vi "Page_Advanced_Initialize.vi"(6 "ctl references":T1, 8 "error in (no error)":errorcluster, 11 "AB_SourceDistribution in":refnum<class "AB_WebService.lvclass">) -> (0 "error out":errorcluster, 3 "AB_SourceDistribution out":refnum<class "AB_WebService.lvclass">)   [LabVIEW 2020, in "AB_WebService.lvclass"]
uses:
  <vilib>/AppBuilder/AB_Classes/WebService/AB_WebService.lvclass
  <resource>/Framework/Providers/Builds/AppBuilder/AB_UI_Page_Advanced_References.ctl
  <vilib>/AppBuilder/AB_Classes/TargetFile/AB_Targetfile.lvclass
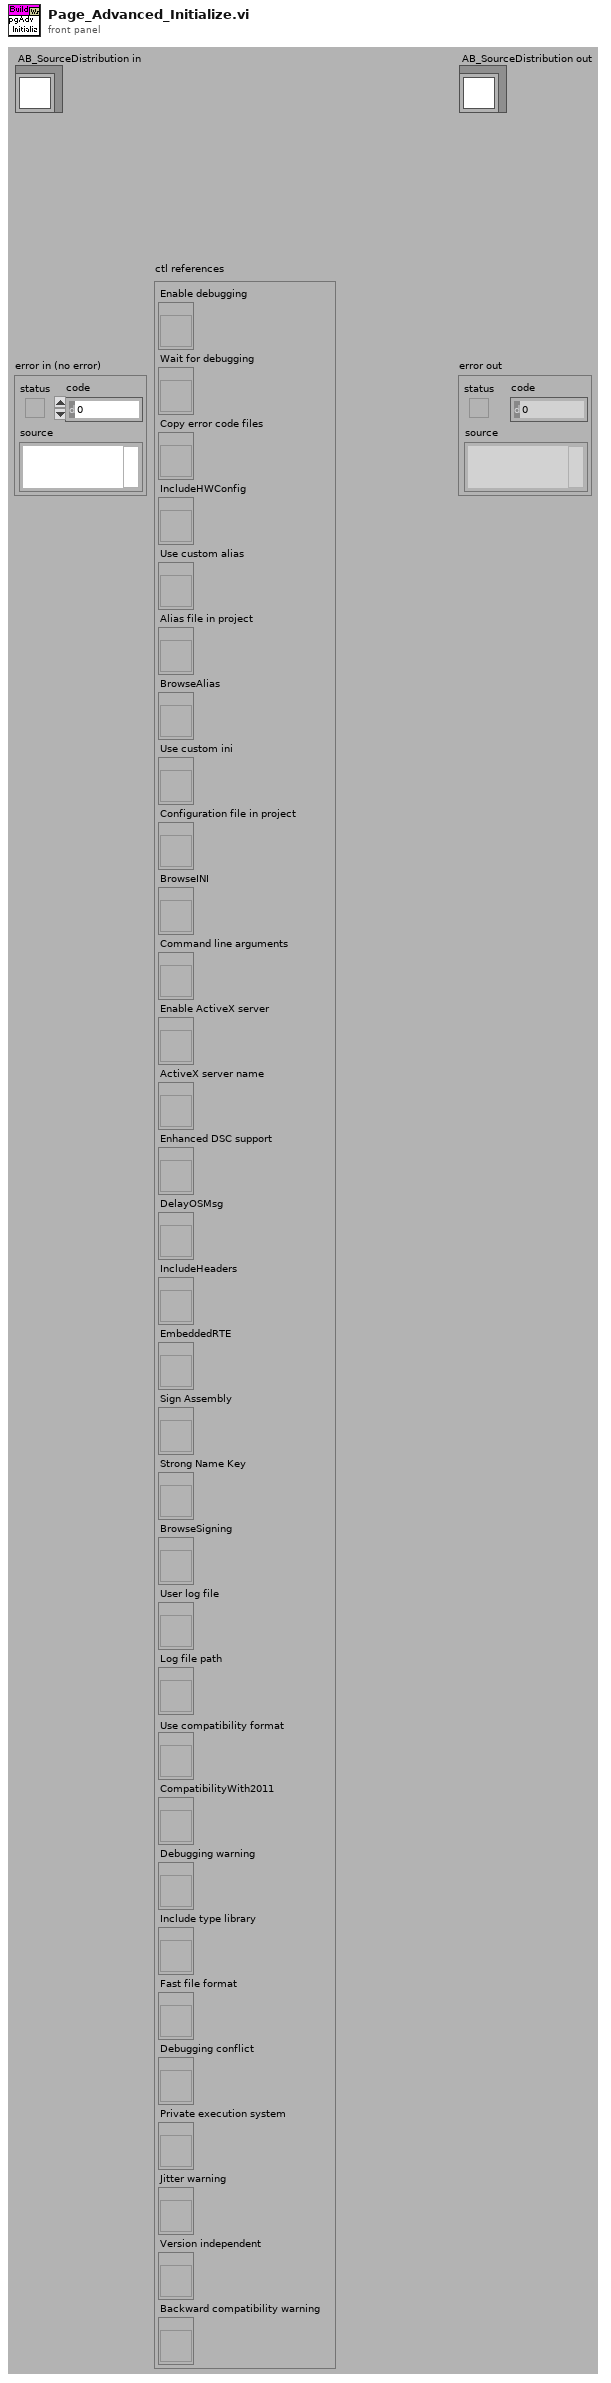
[diagram p1: front panel]
types:
  T1 = typedef "AB_UI_Page_Advanced_References.ctl" = cluster{"Enable debugging":refnum<vi>, "Wait for debugging":refnum<vi>, "Copy error code files":refnum<vi>, "IncludeHWConfig":refnum<vi>, "Use custom alias":refnum<vi>, "Alias file in project":refnum<vi>, "BrowseAlias":refnum<vi>, "Use custom ini":refnum<vi>, "Configuration file in project":refnum<vi>, "BrowseINI":refnum<vi>, "Command line arguments":refnum<vi>, "Enable ActiveX server":refnum<vi>, "ActiveX server name":refnum<vi>, "Enhanced DSC support":refnum<vi>, "DelayOSMsg":refnum<vi>, "IncludeHeaders":refnum<vi>, "EmbeddedRTE":refnum<vi>, "Sign Assembly":refnum<vi>, "Strong Name Key":refnum<vi>, "BrowseSigning":refnum<vi>, "User log file":refnum<vi>, "Log file path":refnum<vi>, "Use compatibility format":refnum<vi>, "CompatibilityWith2011":refnum<vi>, "Debugging warning":refnum<vi>, "Include type library":refnum<vi>, "Fast file format":refnum<vi>, "Debugging conflict":refnum<vi>, "Private execution system":refnum<vi>, "Jitter warning":refnum<vi>, "Version independent":refnum<vi>, "Backward compatibility warning":refnum<vi>}
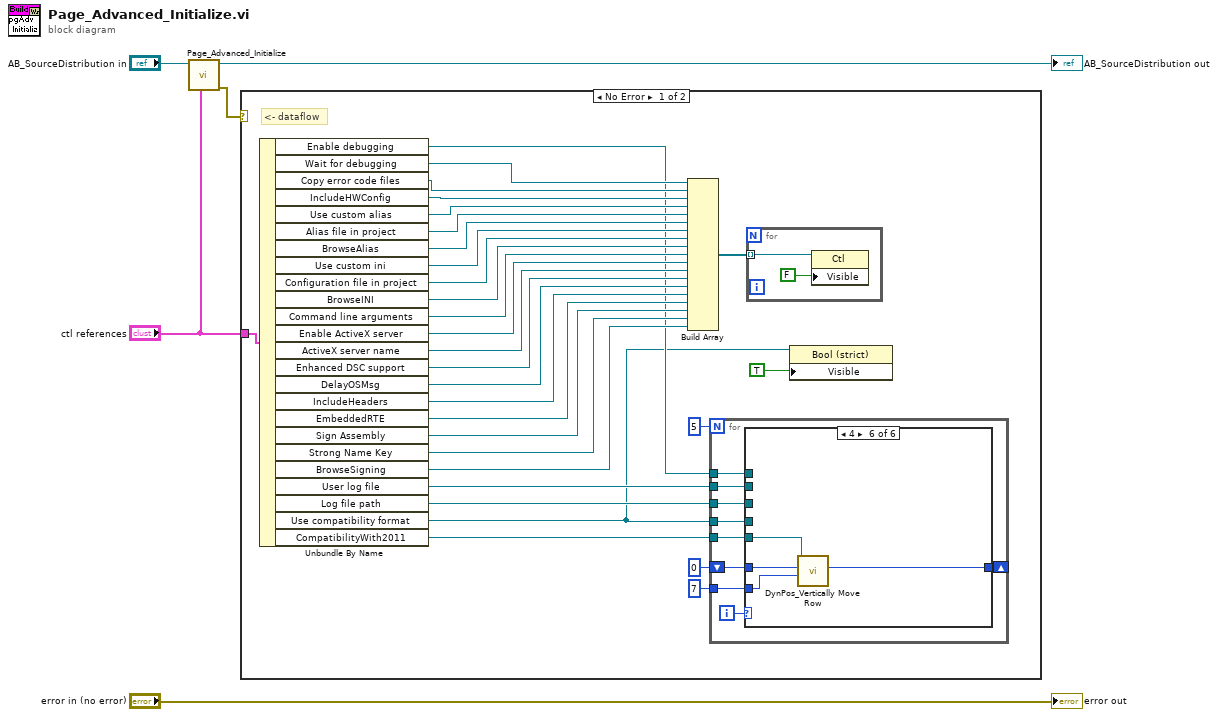
[diagram p0: block diagram]
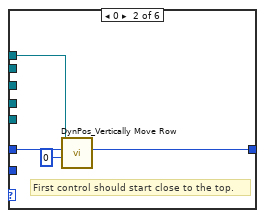
[diagram p3: hidden frame]
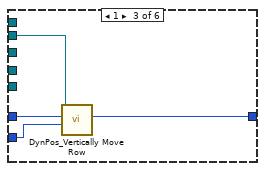
[diagram p4: hidden frame]
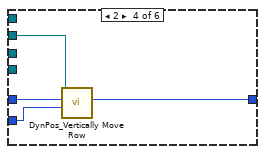
[diagram p5: hidden frame]
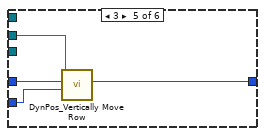
[diagram p6: hidden frame]
diagram:
  n1 = call-parent "Page_Advanced_Initialize.vi"("ctl references"="ctl references", "AB_Build in"="AB_SourceDistribution in") -> ("error out"=w1:errorcluster, "AB_Build out"=→"AB_SourceDistribution out":refnum<class "AB_WebService.lvclass">)  [unwired: 1 in, 7 out]
  n2 = case shown="No Error" w1 {
    tunnel: "ctl references" -> [w35 _]
    frame No Error {
      # "<- dataflow"
      n3 = Unbundle By Name(w35) -> ("Enable debugging"=w9:refnum<vi>, "Wait for debugging"=w34:refnum<vi>, "Copy error code files"=w33:refnum<vi>, "IncludeHWConfig"=w32:refnum<vi>, "Use custom alias"=w31:refnum<vi>, "Alias file in project"=w30:refnum<vi>, "BrowseAlias"=w29:refnum<vi>, "Use custom ini"=w28:refnum<vi>, "Configuration file in project"=w27:refnum<vi>, "BrowseINI"=w26:refnum<vi>, "Command line arguments"=w25:refnum<vi>, "Enable ActiveX server"=w24:refnum<vi>, "ActiveX server name"=w23:refnum<vi>, "Enhanced DSC support"=w22:refnum<vi>, "DelayOSMsg"=w20:refnum<vi>, "IncludeHeaders"=w19:refnum<vi>, "EmbeddedRTE"=w18:refnum<vi>, "Sign Assembly"=w17:refnum<vi>, "Strong Name Key"=w16:refnum<vi>, "BrowseSigning"=w15:refnum<vi>, "User log file"=w13:refnum<vi>, "Log file path"=w12:refnum<vi>, "Use compatibility format"=w7:refnum<vi>, "CompatibilityWith2011"=w6:refnum<vi>)
      n4 = Build Array(w34, w33, w32, w31, w30, w29, w28, w27, w26, w25, w24, w23, w22, w20, w19, w18, w17, w16, w15) -> (w21:refnum<vi>[])
      n5 = for {
        N: 5 -> [_]
        tunnel: w13 -> [w43]
        tunnel: w12 -> [w42]
        shift-right: [w41] -> _
        shift-left: 0 ("Bottom pixel") -> [w40]
        tunnel: 7 ("Bottom pixel") -> [w39]
        tunnel: w9 -> [w38]
        tunnel: w7 -> [w37]
        tunnel: w6 -> [w36]
        i -> [w44]
        n6 = case shown="4" w44 {
          tunnel: w43 -> [_ _ w50 _ _ _]
          tunnel: w42 -> [_ _ _ w54 _ _]
          tunnel: [w45 w48 w53 w57 w61 w65] -> w41
          tunnel: w40 -> [w45 w47 w52 w56 w60 w64]
          tunnel: w39 -> [_ _ w51 w55 w59 w63]
          tunnel: w38 -> [_ w46 _ _ _ _]
          tunnel: w37 -> [_ _ _ _ w58 _]
          tunnel: w36 -> [_ _ _ _ _ w62]
          frame Default {
          }
          frame 0 {
            # "First control should start close to the top."
            n7 = call <vilib>:"DynPos_Vertically Move Row.vi"("Pixel separation (6)"=0, "Bottom of last control"=w47, "Control"=w46) -> ("Bottom pixel"=w48:i32)  [unwired: 1 in, 7 out]
          }
          frame 1 {
            n8 = call <vilib>:"DynPos_Vertically Move Row.vi"("Pixel separation (6)"=w51, "Bottom of last control"=w52, "Control"=w50) -> ("Bottom pixel"=w53:i32)  [unwired: 1 in, 7 out]
          }
          frame 2 {
            n9 = call <vilib>:"DynPos_Vertically Move Row.vi"("Pixel separation (6)"=w55, "Bottom of last control"=w56, "Control"=w54) -> ("Bottom pixel"=w57:i32)  [unwired: 1 in, 7 out]
          }
          frame 3 {
            n10 = call <vilib>:"DynPos_Vertically Move Row.vi"("Pixel separation (6)"=w59, "Bottom of last control"=w60, "Control"=w58) -> ("Bottom pixel"=w61:i32)  [unwired: 1 in, 7 out]
          }
          frame 4 {
            n11 = call <vilib>:"DynPos_Vertically Move Row.vi"("Pixel separation (6)"=w63, "Bottom of last control"=w64, "Control"=w62) -> ("Bottom pixel"=w65:i32)  [unwired: 1 in, 7 out]
          }
        }
      }
      n12 = for {
        tunnel: w21 -> [w67] mode=indexing
        n13 = property class="Ctl"(reference=w67, "Visible"=FALSE) -> ()  [unwired: 1 in, 2 out]
      }
      n14 = property class="Bool (strict)"(reference=w7, "Visible"=TRUE) -> ()  [unwired: 1 in, 2 out]
    }
    frame Error {
    }
  }
  "error out" <- "error in (no error)"
